vi "demo mode.vi"() -> ()   [LabVIEW 2025]
panel:
  out "Demo mode":bool
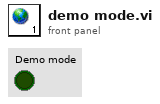
[diagram p1: front panel]
diagram:
